vi "Eat.vi"(8 "error in (no error)":errorcluster, 10 "String":string, 11 "Animal in":refnum<class "Animal.lvclass">) -> (0 "error out":errorcluster, 2 "String 2":string, 3 "Animal out":refnum<class "Animal.lvclass">)   [LabVIEW 2018, in "Animal.lvclass"]
uses:
  Animal.lvclass
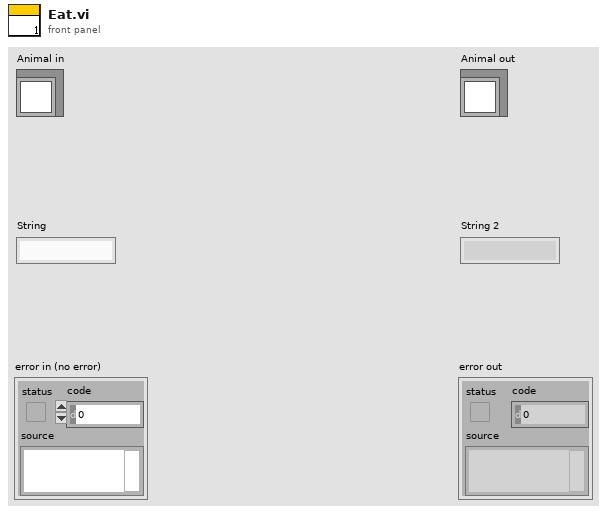
[diagram p1: front panel]
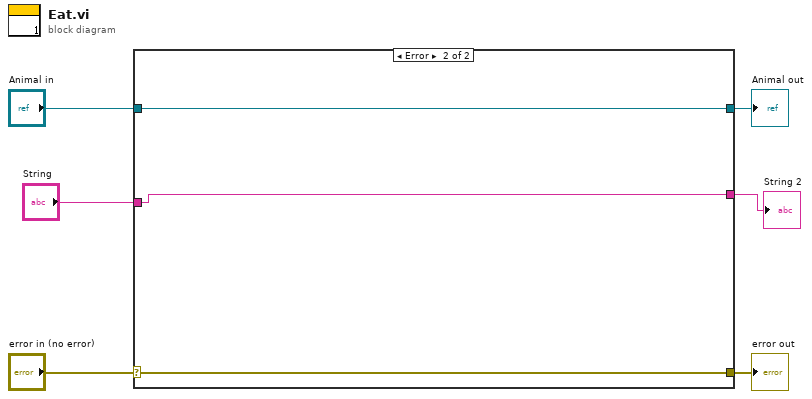
[diagram p0: block diagram]
diagram:
  n1 = case shown="Error" "error in (no error)" {
    selector: "error in (no error)" -> [w8 w12]
    tunnel: [w8 w12] -> w5
    tunnel: [w9 w11] -> w3
    tunnel: "Animal in" -> [w9 w11]
    tunnel: [w7 w10] -> w2
    tunnel: "String" -> [w7 w10]
    frame No Error {
      # "Wire the error cluster across even in the \"No Error\"\ncase so that warnings get propagated."
    }
    frame Error {
    }
  }
  "error out" <- w5
  "Animal out" <- w3
  "String 2" <- w2
